vi "Request Ownership.vi"(8 "error in (no error)":errorcluster, 9 "Shared Resource":bool, 10 "Dependency":refnum<class "SMO.lvclass">, 11 "SMO in":refnum<class "SMO.lvclass">) -> (0 "error out":errorcluster, 2 "Dependency out":refnum<class "SMO.lvclass">, 3 "SMO out":refnum<class "SMO.lvclass">)   [LabVIEW 2021, in "smo.lvlib" / "SMO.lvclass"]
uses:
  SMO.lvclass
  SMO.lvclass/SMO.ctl
  Support/Attribute.Owner/Attribute.Owner.lvclass/Attribute.Owner.ctl
  Support/Attribute.Identity/Attribute.Identity.lvclass/Attribute.Identity.ctl
  Support/Attribute/Attribute.lvclass/Attribute.ctl
  Support/Attribute.Owner/Verify Key Match.vi
  GetVariant(Attr).vi
  Support/Attribute.Identity/Read UniqueName.vi
  Support/Attribute.Identity/Read Given Name.vi
  Support/Attribute.Identity/Read ProspectiveOwner.vi
  Support/Attribute.Owner/Read Lineage.vi
  Support/Attribute/Read AttrName.vi
  ReftoDVR--SMO.vi
  Support/Attribute.Owner/Read Shared Key.vi
  Support/Attribute.Owner/Attribute.Owner.lvclass
  C:/Repositories/SMO/src/Support/Attribute/Attribute.lvclass
  Support/Attribute.SharedResource/Attribute.SharedResource.lvclass
  Support/Attribute.Identity/Attribute.Identity.lvclass
  <vilib>/Utility/MD5Checksum.llb/MD5Checksum string.vi
  <vilib>/Utility/LVClass/Get LV Class Name.vi
  <vilib>/Utility/error.llb/Error Cluster From Error Code.vi
  Support/Attribute/Attribute.lvclass
  Registry/Registry-SMO.lvclass
  C:/Repositories/SMO/src/Support/Attribute.Owner/Attribute.Owner.lvclass
  C:/Repositories/SMO/src/Support/Attribute.Identity/Attribute.Identity.lvclass
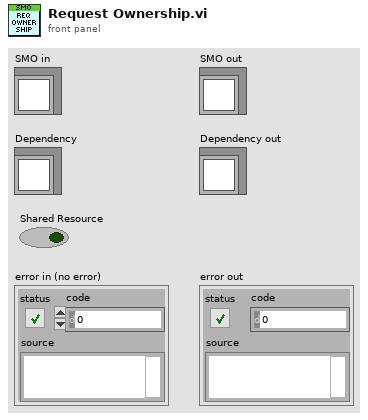
[diagram p1: front panel]
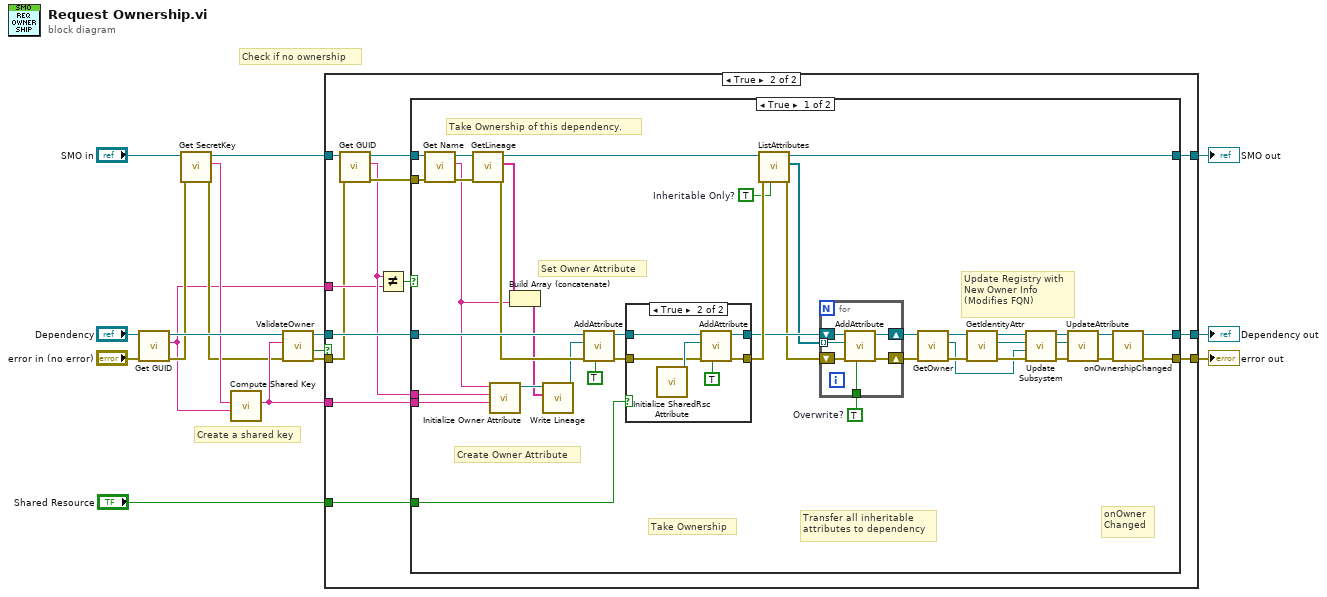
[diagram p0: block diagram]
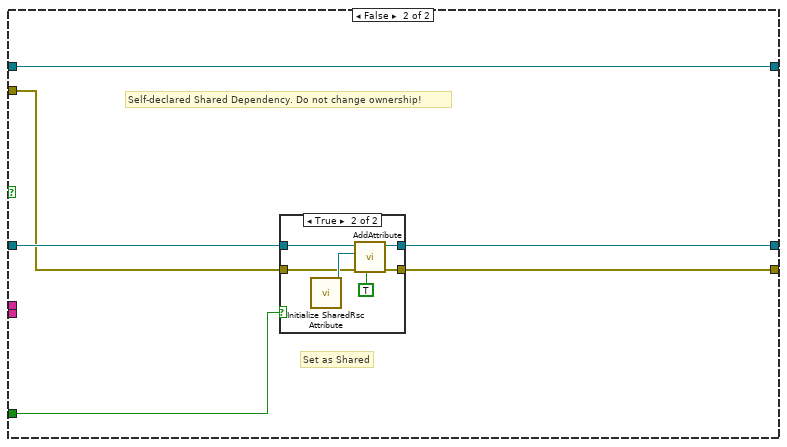
[diagram p4: hidden frame]
diagram:
  # "Check if no ownership"
  # "Create a shared key"
  n1 = call "Get GUID.vi"("error in (no error)"="error in (no error)", "SMO"="Dependency") -> ("error out"=w6:errorcluster, "GUID"=w1:string, "SMO out"=w13:refnum<class "SMO.lvclass">)  [unwired: 7 in]
  n2 = call "Get SecretKey.vi"("error in (no error)"=w6, "SMO"="SMO in") -> ("error out"=w3:errorcluster, "SecretKey"=w5:string, "SMO out"=w4:refnum<class "SMO.lvclass">)  [unwired: 7 in]
  n3 = call "Compute Shared Key.vi"("GUID"=w1, "SecretKey"=w5) -> ("Shared Key"=w15:string)  [unwired: 9 in]
  n4 = call "ValidateOwner.vi"("error in (no error)"=w3, "Shared Key"=w15, "SMO in"=w13) -> ("error out"=w16:errorcluster, "not set"=w2:bool, "SMO out"=w14:refnum<class "SMO.lvclass">)  [unwired: 5 in, 1 out]
  n5 = case shown="True" w2 {
    tunnel: [w20 w30] -> w17
    tunnel: w4 -> [w20 w27]
    tunnel: "Shared Resource" -> [_ w33]
    tunnel: [w19 w29] -> w11
    tunnel: [w18 w28] -> w12
    tunnel: w14 -> [w19 w32]
    tunnel: w15 -> [_ w31]
    tunnel: w16 -> [w18 w21]
    tunnel: w1 -> [_ w23]
    frame False {
      # "Already Owned by other SMO"
    }
    frame True {
      n6 = call "Get GUID.vi"("error in (no error)"=w21, "SMO"=w27) -> ("error out"=w25:errorcluster, "GUID"=w24:string, "SMO out"=w26:refnum<class "SMO.lvclass">)  [unwired: 7 in]
      n7 = Not Equal?(x=w24, y=w23) -> (x != y?=w22:bool)
      n8 = case shown="True" w22 {
        tunnel: w33 -> [w72 w92]
        tunnel: w32 -> [w69 w91]
        tunnel: w31 -> [w68 _]
        tunnel: [w67 w89] -> w30
        tunnel: [w35 w88] -> w29
        tunnel: [w37 w87] -> w28
        tunnel: w26 -> [w50 w89]
        tunnel: w25 -> [w49 w90]
        tunnel: w24 -> [w48 _]
        frame True {
          w62 = TRUE  # Overwrite?
          w65 = TRUE  # Inheritable Only?
          # "onOwner\nChanged"
          # "Update Registry with\nNew Owner Info\n(Modifies FQN)"
          # "Take Ownership of this dependency."
          # "Transfer all inheritable\nattributes to dependency"
          # "Take Ownership"
          # "Create Owner Attribute"
          # "Set Owner Attribute"
          n9 = call "Get Name.vi"("error in (no error)"=w49, "SMO"=w50) -> ("error out"=w57:errorcluster, "Name"=w52:string, "SMO out"=w59:refnum<class "SMO.lvclass">)  [unwired: 5 in, 2 out]
          n10 = call "GetLineage.vi"("error in (no error)"=w57, "SMO in"=w59) -> ("error out"=w56:errorcluster, "Lineage"=w53:string[], "SMO out"=w58:refnum<class "SMO.lvclass">)  [unwired: 7 in]
          n11 = call "Initialize Owner Attribute.vi"("Shared Key"=w68, "Owner GUID"=w48, "Owner Name"=w52) -> ("Attribute.Owner"=w55:refnum<class "Attribute.Owner.lvclass">)  [unwired: 8 in]
          n12 = Build Array (concatenate)(w53, w52) -> (w51:string[])
          n13 = call "Write Lineage.vi"("Lineage"=w51, "Attribute.Owner in"=w55) -> ("Attribute.Owner out"=w54:refnum<class "Attribute.Owner.lvclass">)  [unwired: 8 in, 1 out]
          n14 = call "AddAttribute.vi"("Overwrite? (F)"=TRUE, "error in (no error)"=w56, "Attribute"=w54, "SMO in"=w69) -> ("error out"=w71:errorcluster, "SMO in"=w70:refnum<class "SMO.lvclass">)  [unwired: 6 in]
          n15 = case shown="True" w72 {
            tunnel: w70 -> [w80 w86]
            tunnel: [w80 w85] -> w64
            tunnel: w71 -> [w79 w83]
            tunnel: [w79 w82] -> w66
            frame False {
            }
            frame True {
              n16 = call "Initialize SharedRsc Attribute.vi"() -> ("Attribute.SharedResource"=w84:refnum<class "Attribute.SharedResource.lvclass">)  [unwired: 11 in]
              n17 = call "AddAttribute.vi"("Overwrite? (F)"=TRUE, "error in (no error)"=w83, "Attribute"=w84, "SMO in"=w86) -> ("error out"=w82:errorcluster, "SMO out"=w85:refnum<class "SMO.lvclass">)  [unwired: 6 in]
            }
          }
          n18 = call "ListAttributes.vi"("Inheritable Only? (F: all)"=w65, "error in (no error)"=w66, "SMO in"=w58) -> ("error out"=w63:errorcluster, "[Attributes]"=w61:refnum<class "Attribute.lvclass">[], "SMO out"=w67:refnum<class "SMO.lvclass">)  [unwired: 6 in]
          n19 = for {
            tunnel: w62 -> [w74]
            shift-right: [w78] -> w42
            shift-left: w64 -> [w77]
            shift-right: [w75] -> w40
            shift-left: w63 -> [w76]
            tunnel: w61 -> [w73] mode=indexing
            n20 = call "AddAttribute.vi"("Overwrite? (F)"=w74, "error in (no error)"=w76, "Attribute"=w73, "SMO in"=w77) -> ("error out"=w75:errorcluster, "SMO out"=w78:refnum<class "SMO.lvclass">)  [unwired: 6 in]
          }
          n21 = call "GetOwner.vi"("error in (no error)"=w40, "SMO in"=w42) -> ("error out"=w39:errorcluster, "Owner"=w34:refnum<class "Attribute.Owner.lvclass">, "SMO out"=w41:refnum<class "SMO.lvclass">)  [unwired: 6 in, 1 out]
          n22 = call "GetIdentityAttr.vi"("error in (no error)"=w39, "SMO in"=w41) -> ("error out"=w44:errorcluster, "Attribute.Identity"=w46:refnum<class "Attribute.Identity.lvclass">, "SMO out"=w47:refnum<class "SMO.lvclass">)  [unwired: 7 in]
          n23 = call "Update Subsystem.vi"("error in (no error)"=w44, "New Owner"=w34, "Current Identity"=w46) -> ("error out"=w43:errorcluster, "Updated Identity"=w45:refnum<class "Attribute.Identity.lvclass">)  [unwired: 7 in]
          n24 = call "UpdateAttribute.vi"("error in (no error)"=w43, "Attribute"=w45, "SMO in"=w47) -> ("error out"=w38:errorcluster, "SMO out"=w36:refnum<class "SMO.lvclass">)  [unwired: 6 in, 1 out]
          n25 = call-dynamic "onOwnershipChanged.vi"("error in"=w38, "SMO in"=w36) -> ("error out"=w37:errorcluster, "SMO out"=w35:refnum<class "SMO.lvclass">)  [unwired: 8 in]
        }
        frame False {
          # "Self-declared Shared Dependency. Do not change ownership!"
          # "Set as Shared"
          n26 = case shown="True" w92 {
            tunnel: w91 -> [w94 w100]
            tunnel: [w94 w99] -> w88
            tunnel: w90 -> [w93 w97]
            tunnel: [w93 w96] -> w87
            frame False {
            }
            frame True {
              n27 = call "Initialize SharedRsc Attribute.vi"() -> ("Attribute.SharedResource"=w98:refnum<class "Attribute.SharedResource.lvclass">)  [unwired: 11 in]
              n28 = call "AddAttribute.vi"("Overwrite? (F)"=TRUE, "error in (no error)"=w97, "Attribute"=w98, "SMO in"=w100) -> ("error out"=w96:errorcluster, "SMO out"=w99:refnum<class "SMO.lvclass">)  [unwired: 6 in]
            }
          }
        }
      }
    }
  }
  "SMO out" <- w17
  "error out" <- w12
  "Dependency out" <- w11
